vi "Docteur.vi"() -> ()   [LabVIEW 2016]
uses:
  <vilib>/httpClient/LabVIEWHTTPClient.lvlib
panel:
  in  "String 2":string
  in  "String":string
  in  "?":bool
  out "new picture":picture
  # "Supervision"
  # "Doctor's Id : \n\n   \n    Password :"
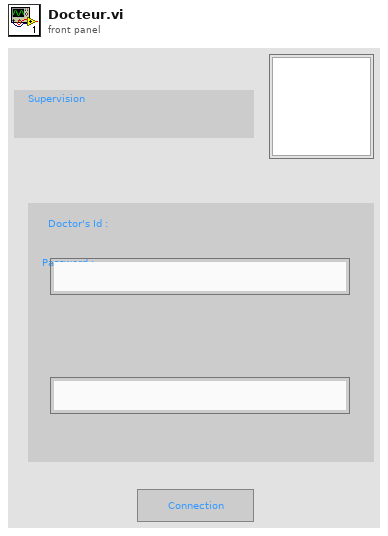
[diagram p1: front panel]
types:
  T1 = typedef "imagedata.ctl" = cluster{"image type":i32, "image depth":i32, "image":u8[], "mask":u8[], "colors":u32[], "Rectangle":cluster{"left":i16, "top":i16, "right":i16, "bottom":i16}}
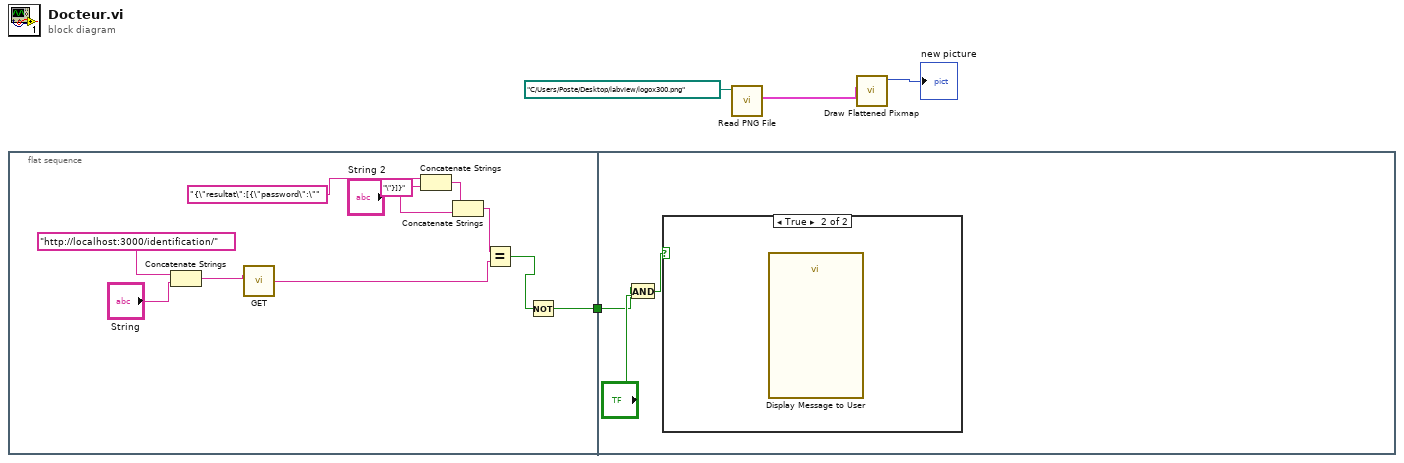
[diagram p0: block diagram]
diagram:
  n1 = flat-sequence {
    tunnel: [w5] -> w1
    tunnel: w1 -> [w16]
    frame #0 {
      n2 = Concatenate Strings("http://localhost:3000/identification/", "String") -> (w14:string)
      n3 = call <vilib>:"GET.vi"("url"=w14) -> ("body"=w8:string)  [unwired: 11 in, 3 out]
      n4 = Concatenate Strings("{\"resultat\":[{\"password\":\"", "String 2") -> (w11:string)
      n5 = Concatenate Strings(w11, "\"}]}") -> (w9:string)
      n6 = Equal?(x=w9, y=w8) -> (x = y?=w6:bool)
      n7 = Not(x=w6) -> (.not. x?=w5:bool)
    }
    frame #1 {
      n8 = And(x=w16, y="?") -> (x .and. y?=w17:bool)
      n9 = case shown="True" w17 {
        frame False {
        }
        frame True {
          n10 = call "Display Message to User"() -> ()  [unwired: 10 in, 2 out]
        }
      }
    }
  }
  n11 = call <vilib>:"Read PNG File.vi"("path to PNG file"=path "C:/Users/Poste/Desktop/labview/logox300.png") -> ("image data"=w3:T1)  [unwired: 8 in, 2 out]
  n12 = call <vilib>:"Draw Flattened Pixmap.vi"("image data"=w3) -> ("new picture"=→"new picture":picture)  [unwired: 8 in]
